vi "shared-dependency-concurrency-test.vi"(8 "error in (no error)":errorcluster) -> (0 "error out":errorcluster)   [LabVIEW 2021]
uses:
  _test-support-SMOs/SMO.A/SMO.A.lvclass
  C:/Repositories/SMO/src/SMO/SMO.lvclass
  src/SMO/SMO.lvclass
  <vilib>/addons/_JKI Toolkits/Caraya/classes/Assert/Assert.lvclass
  <vilib>/addons/_JKI Toolkits/Caraya/classes/Test/Test.lvclass
panel:
  out "size(s) 2":i32
  out "size(s)":i32
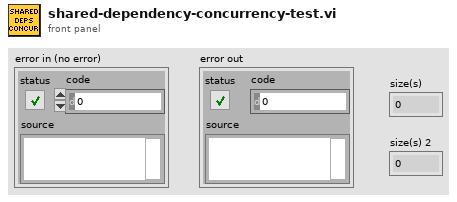
[diagram p1: front panel]
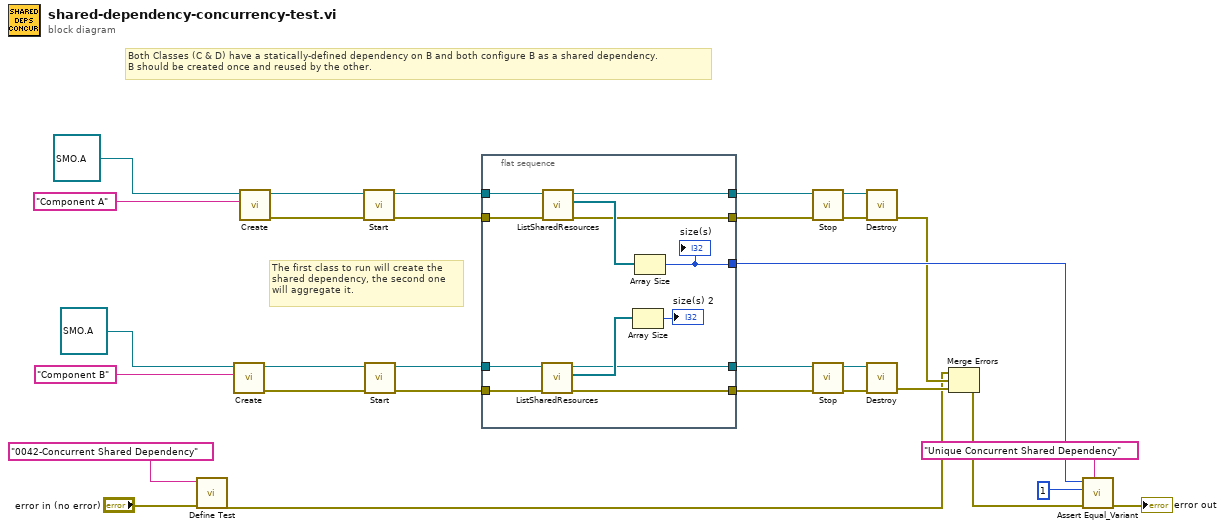
[diagram p0: block diagram]
diagram:
  # "Both Classes (C & D) have a statically-defined dependency on B and both configure B as a shared dependency.\nB should be created once and reused by the other."
  # "The first class to run will create the\nshared dependency, the second one\nwill aggregate it."
  n1 = call <vilib>:"Define Test.vi"("error in (no error)"="error in (no error)", "Label (VI Title)"="0042-Concurrent Shared Dependency") -> ("error out"=w5:errorcluster)  [unwired: 9 in]
  n2 = call "Create.vi"("Subsystem Name (optional)"="Component B", "SMO"=refnum<class "SMO.A.lvclass"> refnum ("SMO.A.lvclass")) -> ("error out"=w6:errorcluster, "SMO out"=w9:refnum<class "SMO.A.lvclass">)  [unwired: 7 in, 1 out]
  n3 = call "Create.vi"("Subsystem Name (optional)"="Component A", "SMO"=refnum<class "SMO.A.lvclass"> refnum ("SMO.A.lvclass")) -> ("error out"=w13:errorcluster, "SMO out"=w19:refnum<class "SMO.A.lvclass">)  [unwired: 7 in, 1 out]
  n4 = call "Start.vi"("error in (no error)"=w13, "SMO"=w19) -> ("error out"=w7:errorcluster, "SMO out"=w24:refnum<class "SMO.A.lvclass">)  [unwired: 8 in]
  n5 = call "Start.vi"("error in (no error)"=w6, "SMO"=w9) -> ("error out"=w12:errorcluster, "SMO out"=w25:refnum<class "SMO.A.lvclass">)  [unwired: 8 in]
  n6 = flat-sequence {
    tunnel: [w42] -> w29
    tunnel: [w40] -> w28
    tunnel: [w32] -> w27
    tunnel: [w34] -> w26
    tunnel: w12 -> [w33]
    tunnel: w25 -> [w35]
    tunnel: w7 -> [w39]
    tunnel: w24 -> [w38]
    tunnel: [w37] -> w15
    frame #0 {
      n7 = call "ListSharedResources.vi"("error in (no error)"=w33, "SMO in"=w35) -> ("error out"=w32:errorcluster, "Shared Resources"=w36:refnum<class "SMO.lvclass">[], "SMO out"=w34:refnum<class "SMO.A.lvclass">)  [unwired: 6 in, 1 out]
      n8 = call "ListSharedResources.vi"("error in (no error)"=w39, "SMO in"=w38) -> ("error out"=w37:errorcluster, "Shared Resources"=w41:refnum<class "SMO.lvclass">[], "SMO out"=w40:refnum<class "SMO.A.lvclass">)  [unwired: 6 in, 1 out]
      n9 = Array Size(array=w36) -> (size(s)=→"size(s) 2":i32)
      n10 = Array Size(array=w41) -> (size(s)=w42:i32)
      "size(s)" <- w42
    }
  }
  n11 = call "Stop.vi"("error in (no error)"=w15, "SMO"=w28) -> ("error out"=w21:errorcluster, "SMO out"=w20:refnum<class "SMO.A.lvclass">)  [unwired: 8 in]
  n12 = call "Stop.vi"("error in (no error)"=w27, "SMO"=w26) -> ("error out"=w10:errorcluster, "SMO out"=w11:refnum<class "SMO.A.lvclass">)  [unwired: 8 in]
  n13 = call "Destroy.vi"("error in (no error)"=w21, "SMO"=w20) -> ("error out"=w23:errorcluster)  [unwired: 9 in]
  n14 = call "Destroy.vi"("error in (no error)"=w10, "SMO"=w11) -> ("error out"=w22:errorcluster)  [unwired: 9 in]
  n15 = Merge Errors(w5, w23, w22) -> (w4:errorcluster)
  n16 = call <vilib>:"Assert Equal_Variant.vi"("Label"="Unique Concurrent Shared Dependency" ("Filter (regex|name)"), "error in (no error)"=w4, "Y"=1, "X"=w29) -> ("error out"=→"error out":errorcluster)  [unwired: 7 in]
